vi "Stop.vi"(8 "error in":errorcluster, 11 "Axis in":refnum<class "Axis.lvclass">) -> (0 "error out":errorcluster, 2 "Success?":bool, 3 "Axis out":refnum<class "Axis.lvclass">)   [LabVIEW 2017, in "Axis.lvlib" / "Axis.lvclass"]
uses:
  Axis.lvclass
  Custom Controls/Command.ctl
  Axis.lvlib
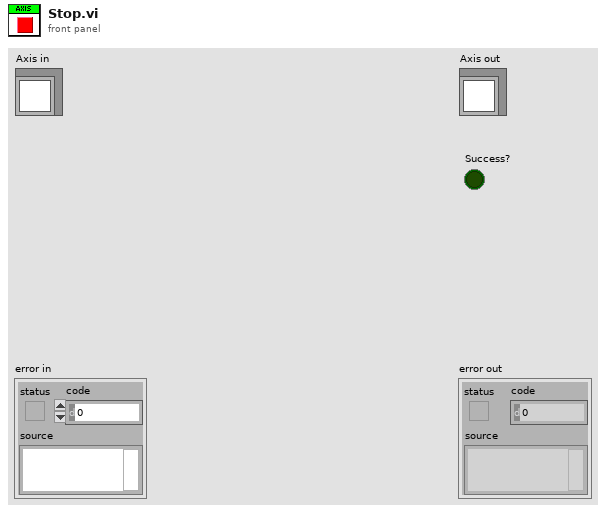
[diagram p1: front panel]
types:
  T1 = typedef "Axis.lvlib/Command.ctl" = enum16{"None", "Home", "Renumber", "Move Absolute", "Move Relative", "Stop", "Set Run Speed", "Set Acceleration", "Set Run Current", "Set Home Offset", "Set Home Speed", "Query Current Position", "Load Defaults", "Query Status", "Lock Controls", "Unlock Controls"}
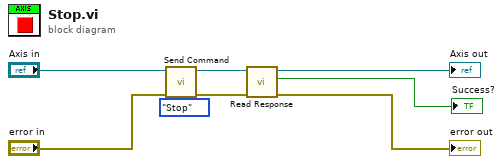
[diagram p0: block diagram]
diagram:
  n1 = call-dynamic "Send Command.vi"("Command"=Command."Stop", "error in (no error)"="error in", "Axis in"="Axis in") -> ("error out"=w5:errorcluster, "Axis out"=w4:refnum<class "Axis.lvclass">)  [unwired: 7 in]
  n2 = call-dynamic "Read Response.vi"("error in (no error)"=w5, "Axis in"=w4) -> ("error out"=→"error out":errorcluster, "Success?"=→"Success?":bool, "Axis out"=→"Axis out":refnum<class "Axis.lvclass">)  [unwired: 7 in]
